vi "GetHelp.vi"(11 "VIPMUninstallPackage in":refnum<class "VIPMUninstallPackage.lvclass">) -> (2 "Help":string, 3 "VIPMUninstallPackage out":refnum<class "VIPMUninstallPackage.lvclass">)   [LabVIEW 2014, in "VIPMUninstallPackage.lvclass"]
uses:
  <nishared>/LabVIEW CLI/Operations/VIPMUninstallPackage/VIPMUninstallPackage.lvclass
panel:
  in  "Help":string="LabVIEWCLI -OperationName VIPMUninstallPackage -PackageName <package name> -LabVIEWVersion <labview version string>\n\n -PackageName: Specifies the name of the VIPM package to install (e.g. package_abc_api-2.5.0.0)\n\n -LabVIEWVersion : Specifies the version of LabVIEW to uninstall the VIPM package from (e.g. \"17.0\", \"17.0 (64-bit)\", \"18.0\", \"18.0 (64-bit)\", ...)\n\nNote: You must have the VIPM API installed and have a JKI VI Package Manager Pro license.\n"
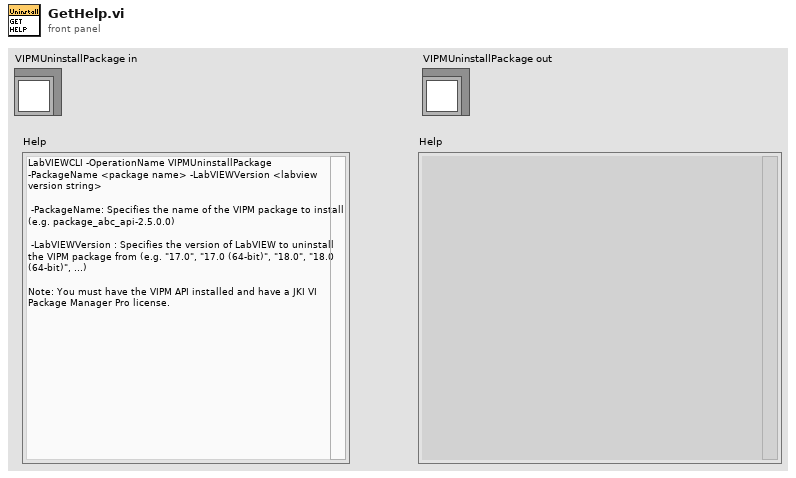
[diagram p1: front panel]
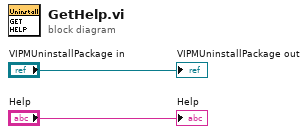
[diagram p0: block diagram]
diagram:
  "VIPMUninstallPackage out" <- "VIPMUninstallPackage in"
  "Help" <- "Help"
